vi "GetAttributeViReal64_ACP_CL_DD.vi"(8 "error in (no error)":errorcluster {"code" format="%.0x"}, 9 "AttributeID":u32(ring)=1150014 items=["ACP_CARRIER_CPSD"=1150014, "ACP_CARRIER_REFERENCE_FREQUENCY"=1150015, "ACP_CARRIER_REFERENCE_LEVEL"=1150017, "ACP_DISPLAY_WINDOWY_REFERENCE"=1150091, "ACP_DISPLAY_WINDOWY_SCALE"=1150092, "ACP_FREQUENCY_SPAN"=1150094, "ACP_INTEGRATION_BANDWIDTH"=1191694, "ACP_MARKER_AMPLITUDE"=1150096, "ACP_MARKER_POSITION"=1150101, "ACP_MARKER_TRACE_POINTS_POSITION"=1190657, "ACP_OFFSET_FILTER_ALPHA"=1150103, "ACP_SWEEPCOUPLING_RESOLUTION_BANDWIDTH"=1150023, "ACP_SWEEPCOUPLING_SWEEP_TIME"=1150027, "ACP_SWEEPCOUPLING_VIDEO_BANDWIDTH"=1150030, "APERTURE"=1191708, "DIGITAL_DEMOD_ADJUST_CLOCK"=1191641, "DIGITAL_DEMOD_APSK_RING2_RATIO"=1191631, "DIGITAL_DEMOD_APSK_RING3_RATIO"=1191632, "DIGITAL_DEMOD_DISPLAY_IDEAL_STATE_SIZE"=1191616, "DIGITAL_DEMOD_DISPLAY_WINDOW_X_REFERENCE"=1191609, "DIGITAL_DEMOD_DISPLAY_WINDOW_X_WIDTH"=1191658, "DIGITAL_DEMOD_DISPLAY_WINDOW_Y_REFERENCE"=1191591, "DIGITAL_DEMOD_DISPLAY_WINDOW_Y_SCALE"=1191590, "DIGITAL_DEMOD_EQUALIZATION_CONVERGENCE"=1191636, "DIGITAL_DEMOD_FILTER_ALPHA"=1191628, "DIGITAL_DEMOD_FILTER_BETA"=1191629, "DIGITAL_DEMOD_FSK_DEVIATION_REFERENCE"=1191638, "DIGITAL_DEMOD_FSK_TX_FREQUENCY_OFFSET"=1191640, "DIGITAL_DEMOD_IQ_ROTATION"=1191664, "DIGITAL_DEMOD_LIMITS_CLOCK_ERROR_IN_HERTZ"=1191619, "DIGITAL_DEMOD_LIMITS_CLOCK_ERROR_INPPM"=1191622, "DIGITAL_DEMOD_LIMITS_DEVIATION_ACCURACY"=1191647, "DIGITAL_DEMOD_LIMITS_FREQUENCY_ERROR_IN_HERTZ"=1191618, "DIGITAL_DEMOD_LIMITS_FREQUENCY_ERROR_INPPM"=1191623, "DIGITAL_DEMOD_LIMITS_POWER_LIMIT"=1191624, "DIGITAL_DEMOD_LIMITS_RMS_FSK_ERROR"=1191646, "DIGITAL_DEMOD_LIMITS_RMS_OFFSETEVM"=1191648, "DIGITAL_DEMOD_MARKER_AMPLITUDE"=1191594, "DIGITAL_DEMOD_MARKER_FUNCTION_BAND_LEFT"=1191602, "DIGITAL_DEMOD_MARKER_FUNCTION_BAND_RIGHT"=1191603, "DIGITAL_DEMOD_MARKER_FUNCTION_BAND_SPAN"=1191604, "DIGITAL_DEMOD_MARKER_POSITION"=1191599, "DIGITAL_DEMOD_MARKER_WINDOW_TRACE"=1191681, "DIGITAL_DEMOD_MARKER_Y_IMAGINARY"=1191682, "DIGITAL_DEMOD_MULTI_CARRIER_FILTER_BANDWIDTH"=1191680, "DIGITAL_DEMOD_SAMPLE_RATE"=1191617, "DIGITAL_DEMOD_SWEEP_COUPLING_RESOLUTION_BANDWIDTH"=1191762, "DIGITAL_DEMOD_SYMBOL_INTERVAL"=1191659, "DIGITAL_DEMOD_SYNC_BURST_SEARCH_THRESHOLD"=1191652, "DIGITAL_DEMOD_SYNC_SEARCH_LENGTH"=1191653, "DIGITAL_DEMOD_TRACE_LIMIT_MARGIN"=1191674, "DIGITAL_DEMOD_TRACE_LIMIT_X_OFFSET"=1191673, "DIGITAL_DEMOD_TRACE_LIMIT_Y_OFFSET"=1191760, "FREQUENCY_CENTER_STEP"=1150133, "FREQUENCY_CENTER"=1190114, "GATING_DELAY"=1190014, "GATING_HOLD_OFF_TIME"=1150142, "GATING_LENGTH"=1190016, "GATING_MIN_FAST"=1190017, "GATING_VIEW_START_TIME"=1191460, "GATING_VIEW_SWEEP_TIME"=1190021, "INPUT_IQ_CENTER_FREQUENCY"=1191715, "INPUT_IQ_I_ATTENUATION"=1190851, "INPUT_IQ_I_ATTENUATION_RATIO"=1190853, "INPUT_IQ_I_EXTERNAL_GAIN"=1190840, "INPUT_IQ_I_OFFSET"=1191697, "INPUT_IQ_I_SKEW_FACTOR"=1190843, "INPUT_IQ_Q_ATTENUATION_RATIO"=1190854, "INPUT_IQ_Q_ATTENUATION"=1190852, "INPUT_IQ_Q_EXTERNAL_GAIN"=1190841, "INPUT_IQ_Q_OFFSET"=1191698, "INPUT_IQ_Q_SKEW_FACTOR"=1190842, "INPUT_IQ_REFERENCE_IMPEDANCE"=1191700, "INPUT_RF_BASE_STATION_GAIN"=1190115, "INPUT_RF_MOBILE_STATION_GAIN"=1190116, "LEVEL_ATTENUATION"=1190002, "LEVEL_ELECTRONIC_ATTENUATION"=1190121], 10 "RepCapIdentifier":string, 11 "instrument handle":refnum<k15>) -> (0 "error out":errorcluster {"code" format="%.0x"}, 2 "AttributeValue":dbl, 3 "instrument handle out":refnum<k15>)   [LabVIEW 2021, in "Keysight XSAnVMA.lvlib"]
doc: "Gets Real64 Attribute from instrumrnt driver.\nThe following attributes are supported:\n\nACP_CARRIER_CPSD\nACP_CARRIER_REFERENCE_FREQUENCY\nACP_CARRIER_REFERENCE_LEVEL\nACP_DISPLAY_WINDOWY_REFERENCE\nACP_DISPLAY_WINDOWY_SCALE\nACP_FREQUENCY_SPAN\nACP_INTEGRATION_BANDWIDTH\nACP_MARKER_AMPLITUDE\nACP_MARKER_POSITION\nACP_MARKER_TRACE_POINTS_POSITION\nACP_OFFSET_FILTER_ALPHA\nACP_SWEEPCOUPLING_RESOLUTION_BANDWIDTH\nACP_SWEEPCOUPLING_SWEEP_TIME\nACP_SWEEPCOUPLING_VIDEO_BANDWIDTH\nAPERTURE\nDIGITAL_DEMOD_ADJUST_CLOCK\nDIGITAL_DEMOD_APSK_RING2_RATIO\nDIGITAL_DEMOD_APSK_RING3_RATIO\nDIGITAL_DEMOD_DISPLAY_IDEAL_STATE_SIZE\nDIGITAL_DEMOD_DISPLAY_WINDOW_X_REFERENCE\nDIGITAL_DEMOD_DISPLAY_WINDOW_X_WIDTH\nDIGITAL_DEMOD_DISPLAY_WINDOW_Y_REFERENCE\nDIGITAL_DEMOD_DISPLAY_WINDOW_Y_SCALE\nDIGITAL_DEMOD_EQUALIZATION_CONVERGENCE\nDIGITAL_DEMOD_FILTER_ALPHA\nDIGITAL_DEMOD_FILTER_BETA\nDIGITAL_DEMOD_FSK_DEVIATION_REFERENCE\nDIGITAL_DEMOD_FSK_TX_FREQUENCY_OFFSET\nDIGITAL_DEMOD_IQ_ROTATION\nDIGITAL_DEMOD_LIMITS_CLOCK_ERROR_IN_HERTZ\nDIGITAL_DEMOD_LIMITS_CLOCK_ERROR_INPPM\nDIGITAL_DEMOD_LIMITS_DEVIATION_ACCURACY\nDIGITAL_DEMOD_LIMITS_FREQUENCY_ERROR_IN_HERTZ\nDIGITAL_DEMOD_LIMITS_FREQUENCY_ERROR_INPPM\nDIGITAL_DEMOD_LIMITS_POWER_LIMIT\nDIGITAL_DEMOD_LIMITS_RMS_FSK_ERROR\nDIGITAL_DEMOD_LIMITS_RMS_OFFSETEVM\nDIGITAL_DEMOD_MARKER_AMPLITUDE\nDIGITAL_DEMOD_MARKER_FUNCTION_BAND_LEFT\nDIGITAL_DEMOD_MARKER_FUNCTION_BAND_RIGHT\nDIGITAL_DEMOD_MARKER_FUNCTION_BAND_SPAN\nDIGITAL_DEMOD_MARKER_POSITION\nDIGITAL_DEMOD_MARKER_WINDOW_TRACE\nDIGITAL_DEMOD_MARKER_Y_IMAGINARY\nDIGITAL_DEMOD_MULTI_CARRIER_FILTER_BANDWIDTH\nDIGITAL_DEMOD_SAMPLE_RATE\nDIGITAL_DEMOD_SWEEP_COUPLING_RESOLUTION_BANDWIDTH\nDIGITAL_DEMOD_SYMBOL_INTERVAL\nDIGITAL_DEMOD_SYNC_BURST_SEARCH_THRESHOLD\nDIGITAL_DEMOD_SYNC_SEARCH_LENGTH\nDIGITAL_DEMOD_TRACE_LIMIT_MARGIN\nDIGITAL_DEMOD_TRACE_LIMIT_X_OFFSET\nDIGITAL_DEMOD_TRACE_LIMIT_Y_OFFSET\nFREQUENCY_CENTER_STEP\nFREQUENCY_CENTER\nGATING_DELAY\nGATING_HOLD_OFF_TIME\nGATING_LENGTH\nGATING_MIN_FAST\nGATING_VIEW_START_TIME\nGATING_VIEW_SWEEP_TIME\nINPUT_IQ_CENTER_FREQUENCY\nINPUT_IQ_I_ATTENUATION\nINPUT_IQ_I_ATTENUATION_RATIO\nINPUT_IQ_I_EXTERNAL_GAIN\nINPUT_IQ_I_OFFSET\nINPUT_IQ_I_SKEW_FACTOR\nINPUT_IQ_Q_ATTENUATION_RATIO\nINPUT_IQ_Q_ATTENUATION\nINPUT_IQ_Q_EXTERNAL_GAIN\nINPUT_IQ_Q_OFFSET\nINPUT_IQ_Q_SKEW_FACTOR\nINPUT_IQ_REFERENCE_IMPEDANCE\nINPUT_RF_BASE_STATION_GAIN\nINPUT_RF_MOBILE_STATION_GAIN\nLEVEL_ATTENUATION\nLEVEL_ELECTRONIC_ATTENUATION"
uses:
  <instrlib>/Keysight XSAnVMA/Keysight XSAnVMA.lvlib
  KtXSAnVMA_64.dll
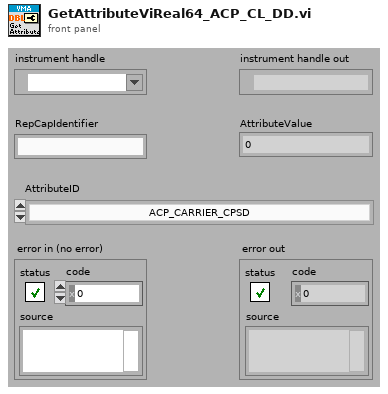
[diagram p1: front panel]
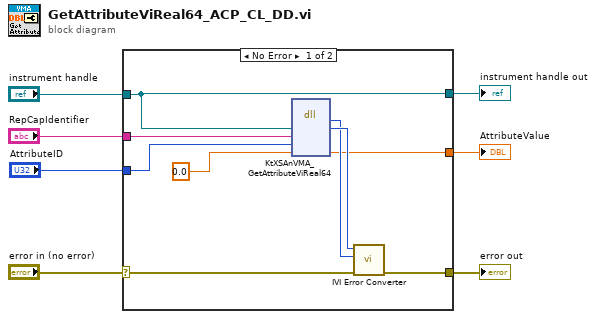
[diagram p0: block diagram]
diagram:
  n1 = case shown="No Error" "error in (no error)" {
    selector: "error in (no error)" -> [w14 w18]
    tunnel: [w13 w18] -> w7
    tunnel: "instrument handle" -> [w8 w17]
    tunnel: "RepCapIdentifier" -> [w12 _]
    tunnel: "AttributeID" -> [w11 _]
    tunnel: [w9 _] -> w3
    tunnel: [w8 w17] -> w2
    frame No Error {
      n2 = dll-call lib="KtXSAnVMA**.dll" fn="KtXSAnVMA_GetAttributeViReal64"("Vi"=w8, "RepCapIdentifier"=w12, "AttributeID"=w11, "AttributeValue"=0.0) -> ("return type"=w15:i32, "Vi"=w16:u32, "AttributeValue"=w9:dbl)  [unwired: 5 in, 2 out]
      n3 = call <instrlib>:"IVI Error Converter.vi"("error in (no error)"=w14, "IVI error code (0)"=w15, "instrument handle"=w16) -> ("error out"=w13:errorcluster)  [unwired: 7 in, 1 out]
    }
    frame Error {
    }
  }
  "error out" <- w7
  "instrument handle out" <- w2
  "AttributeValue" <- w3
